vi "App_Main Initialize.vi"(8 "error in":errorcluster, 10 "Subpanel":refnum<vi>, 11 "VI Reference":refnum<vi>) -> (0 "error out":errorcluster, 3 "Event Registration Refnum":refnum<event-registration>)   [LabVIEW 2018, in "Application 1.lvlib"]
uses:
  Application 1.lvlib
  Data Def/App_User Event Data.ctl
  Cloud Server/Data Def/Server_Error Handle Method.ctl
  Data Def/App_FGV Method.ctl
  Data Def/App_Main Data.ctl
  Com VIs/Data Def/stm_MetaElement.ctl
  Com VIs/Data Def/stm_MetaDataElement.ctl
  Data Def/App_Main Queue.ctl
  Data Def/App_Main Loop Queue Data.ctl
  Com VIs/Data Def/User Data.ctl
  Data Def/App_Config Method.ctl
  Data Def/App_User Event Method.ctl
  Data Def/App_Subpanel Name.ctl
  Cloud Server/Cloud Server.lvlib
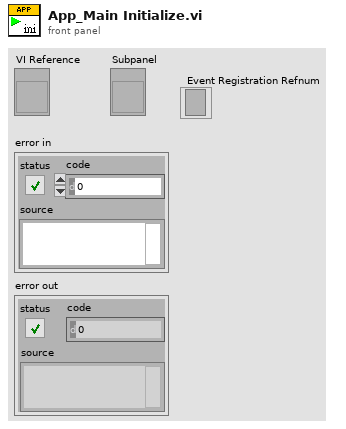
[diagram p1: front panel]
types:
  T1 = typedef "Cloud Server.lvlib/Server_Error Handle Method.ctl" = enum16{"Initialize", "Get Queue Ref.", "Enqueue", "Insert", "Flush", "Release"}
  T2 = typedef "Application 1.lvlib/App_Main Data.ctl" = cluster{"VI Refnum":refnum<vi>, "Subpanel":refnum<vi>, "Connection ID":refnum<k5>, "Meta data":T3[], "Main Queue":T5, "User Data":T6}
  T3 = typedef "stm_MetaElement.ctl" = cluster{"Name":T4}
  T4 = typedef "stm_MetaDataElement.ctl" = string
  T5 = typedef "Application 1.lvlib/App_Main Queue.ctl" = cluster{"Main Loop Queue":refnum<queue>}
  T6 = typedef "User Data.ctl" = cluster{"Name":string, "Email":string, "Phone Number":string, "User Picture":u32[][], "Last Login Time":timestamp}
  T7 = typedef "Application 1.lvlib/App_FGV Method.ctl" = enum16{"Get", "Put"}
  T8 = typedef "Application 1.lvlib/App_Config Method.ctl" = enum16{"Get", "Put", "Load", "Save"}
  T9 = typedef "Application 1.lvlib/App_Subpanel Name.ctl" = enum16{"Main", "Menu", "User Registering", "User Setting", "Monitor", "Traning Mode", "Query Data", "Connect Setting"}
  T10 = typedef "Application 1.lvlib/App_User Event Method.ctl" = enum16{"Initialize", "Put Event", "Get Ref.", "Release"}
  T11 = typedef "Application 1.lvlib/App_Main Loop Queue Data.ctl" = cluster{"Command":string, "Data":variant}
  T12 = typedef "Application 1.lvlib/App_User Event Data.ctl" = cluster{"Command":string, "Data":variant}
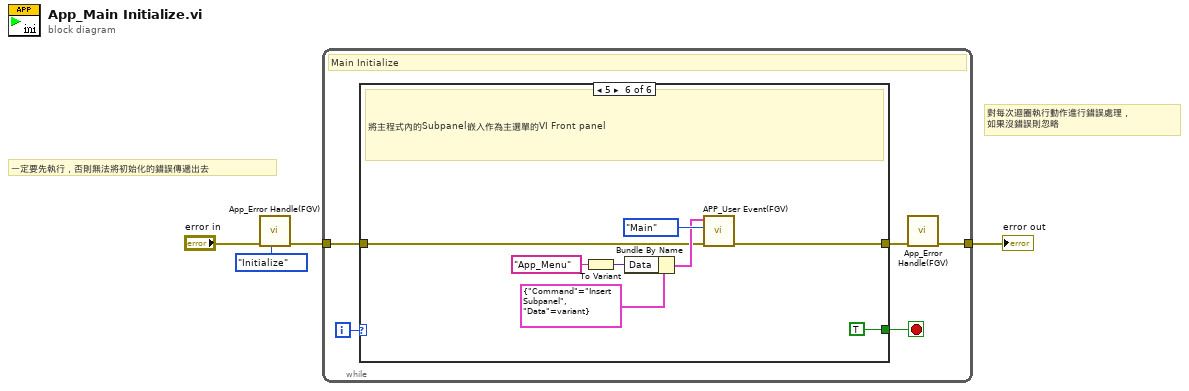
[diagram p0: block diagram]
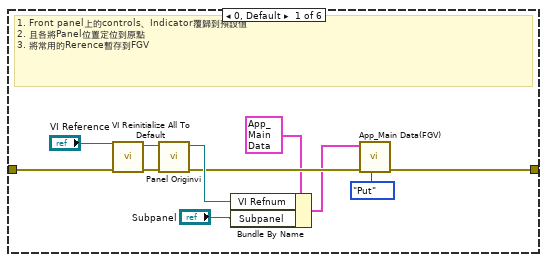
[diagram p2: hidden frame]
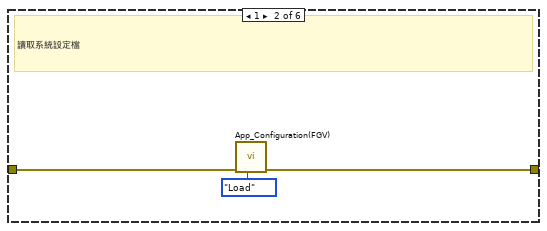
[diagram p3: hidden frame]
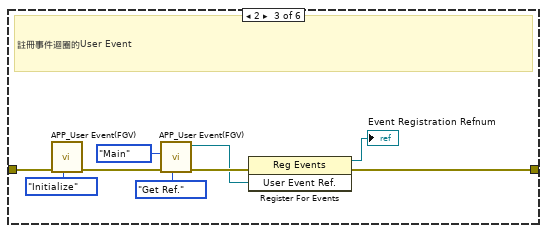
[diagram p4: hidden frame]
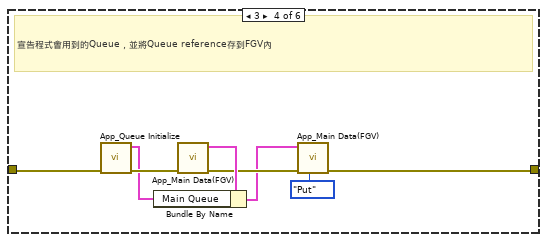
[diagram p5: hidden frame]
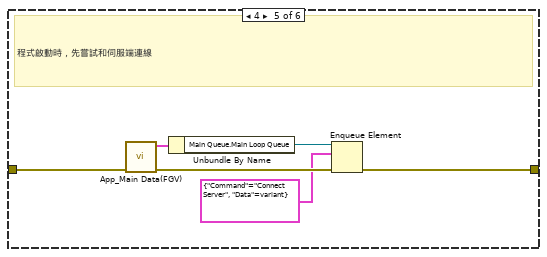
[diagram p6: hidden frame]
diagram:
  # "對每次迴圈執行動作進行錯誤處理，\n如果沒錯誤則忽略"
  # "一定要先執行，否則無法將初始化的錯誤傳遞出去"
  n1 = call "App_Error Handle(FGV).vi"("Error Handle Method(Enqueue)"=Server_Error_Handle_Method."Initialize", "error in"="error in") -> ("error out"=w2:errorcluster)  [unwired: 8 in, 1 out]
  n2 = while {
    tunnel: w2 -> [w8]
    tunnel: [w6] -> w1
    i -> [w9]
    stop <- w5 stop-if-true
    # "Main Initialize"
    n3 = case shown="5" w9 {
      tunnel: w8 -> [w19 w23 w25 w34 w42 w49]
      tunnel: [w14 w22 w24 w33 w41 w48] -> w7
      tunnel: [_ _ _ _ _ TRUE] -> w5
      frame 0, Default {
        # "1. Front panel上的controls、Indicator覆歸到預設值\n2. 且各將Panel位置定位到原點\n3. 將常用的Rerence暫存到FGV"
        n4 = call "VI Reinitialize All To Default.vi"("error in"=w19, "VI Reference in"="VI Reference") -> ("error out"=w20:errorcluster, "VI Reference out"=w17:refnum<vi>)  [unwired: 8 in]
        n5 = call "Panel Originvi.vi"("error in"=w20, "VI Reference In"=w17) -> ("error out"=w12:errorcluster, "VI Reference Out"=w16:refnum<vi>)  [unwired: 8 in]
        n6 = Bundle By Name(cluster=T2 {"VI Refnum"=refnum, "Subpanel"=refnum, "Connection ID"=refnum, "Meta data"=[], "Main Queue"={"Main Loop Queue"=refnum}, "User Data"={"Name"="", "Email"="", "Phone Number"="", "User Picture"=array225x225[50625 elements], "Last Login Time"=timestamp(0 s since 1904-01-01)}} ("Main Data In"), "VI Refnum"=w16, "Subpanel"="Subpanel") -> (w10:T2)
        n7 = call "App_Main Data(FGV).vi"("FGV Method"=App_FGV_Method."Put", "error in"=w12, "Main Data In"=w10) -> ("error out"=w14:errorcluster)  [unwired: 7 in, 1 out]
      }
      frame 1 {
        # "讀取系統設定檔"
        n8 = call "App_Configuration(FGV).vi"("Config Method(Get)"=App_Config_Method."Load", "error in"=w23) -> ("error out"=w22:errorcluster)  [unwired: 8 in, 1 out]
      }
      frame 2 {
        # "註冊事件迴圈的User Event"
        n9 = call "APP_User Event(FGV).vi"("User Event Method(Put Event)"=App_User_Event_Method."Initialize" ("User Event Method"), "error in"=w25) -> ("error out"=w30:errorcluster)  [unwired: 8 in, 1 out]
        n10 = call "APP_User Event(FGV).vi"("User Event Method(Put Event)"=App_User_Event_Method."Get Ref." ("User Event Method"), "error in"=w30, "Subpanel Name"=App_Subpanel_Name."Main") -> ("error out"=w28:errorcluster, "User Event Ref."=w27:refnum<user-event>)  [unwired: 7 in]
        n11 = register-events(error in=w28, w27) -> (reference out=→"Event Registration Refnum":refnum<event-registration>, error out=w24:errorcluster)  [unwired: 1 in]
      }
      frame 3 {
        # "宣告程式會用到的Queue，並將Queue reference存到FGV內"
        n12 = call "App_Queue Initialize.vi"("error in"=w34) -> ("error out"=w40:errorcluster, "Main Queue"=w38:T5)  [unwired: 9 in]
        n13 = call "App_Main Data(FGV).vi"("error in"=w40) -> ("error out"=w37:errorcluster, "Main Data Out"=w39:T2)  [unwired: 9 in]
        n14 = Bundle By Name(cluster=w39, "Main Queue"=w38) -> (w35:T2)
        n15 = call "App_Main Data(FGV).vi"("FGV Method"=App_FGV_Method."Put", "error in"=w37, "Main Data In"=w35) -> ("error out"=w33:errorcluster)  [unwired: 7 in, 1 out]
      }
      frame 4 {
        # "程式啟動時，先嘗試和伺服端連線"
        n16 = call "App_Main Data(FGV).vi"("error in"=w42) -> ("error out"=w45:errorcluster, "Main Data Out"=w46:T2)  [unwired: 9 in]
        n17 = Unbundle By Name(w46) -> ("Main Queue.Main Loop Queue"=w44:refnum<queue>)
        n18 = Enqueue Element(queue=w44, element=T11 {"Command"="Connect Server", "Data"=variant}, error in (no error)=w45) -> (error out=w41:errorcluster)  [unwired: 1 in, 2 out]
      }
      frame 5 {
        # "將主程式內的Subpanel嵌入作為主選單的VI Front panel"
        n19 = To Variant(anything="App_Menu") -> (Variant=w52:variant)
        n20 = Bundle By Name(cluster=T12 {"Command"="Insert Subpanel", "Data"=variant} ("User Event Data"), "Data"=w52) -> (w50:T12)
        n21 = call "APP_User Event(FGV).vi"("error in"=w49, "Subpanel Name"=App_Subpanel_Name."Main", "User Event Data"=w50) -> ("error out"=w48:errorcluster)  [unwired: 7 in, 1 out]
      }
    }
    n22 = call "App_Error Handle(FGV).vi"("error in"=w7) -> ("error out"=w6:errorcluster)  [unwired: 9 in, 1 out]
  }
  "error out" <- w1
